vi "Probe (U64).vi"(9 "Data Valid":bool, 10 "Input Data":u64) -> (1 "Address":u64, 2 "Collected Data":u64[](array[numeric]))   [LabVIEW 2012]
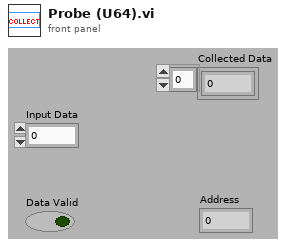
[diagram p1: front panel]
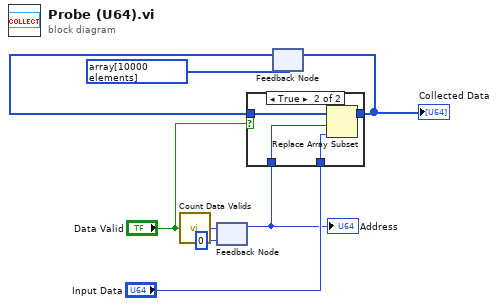
[diagram p0: block diagram]
diagram:
  n1 = call <userlib>:"Count Data Valids.vi"("Data Valid"="Data Valid") -> ("Counter"=w8:u64)  [unwired: 14 in]
  n2 = feedback-in #1(w8) -> ()
  n3 = feedback #1(u64 0 ("Counter")) -> (w2:u64)
  "Address" <- w2
  n4 = feedback #2(u64[] array[10000 elements]) -> (w7:u64[])
  n5 = case shown="True" "Data Valid" {
    tunnel: w2 -> [_ w13]
    tunnel: w7 -> [w9 w12]
    tunnel: [w9 w11] -> w5
    tunnel: "Input Data" -> [_ w10]
    frame False {
    }
    frame True {
      n6 = Replace Array Subset(array=w12, new element=w10, index=w13) -> (w11:u64[])
    }
  }
  "Collected Data" <- w5
  n7 = feedback-in #2(w5) -> ()
